vi "BeamProfile_Proc.vi"(5 "Output filepath (For Type Only)":path=path "", 7 "Params.":variant, 8 "error in (no error)":errorcluster, 9 "Dynamic Params queue":refnum<queue>, 10 "Quit_UserEvent":refnum<user-event>, 11 "ControlQueueRef":variant) -> (0 "error out":errorcluster, 2 "Output":variant)   [LabVIEW 2013]
uses:
  Apps_static/ScanParams_SingleLine.ctl
  Files/BinaryHeader.ctl
  ControlDef/QueueRefs.ctl
  ControlDef/LaserCtrl_Method.ctl
  ControlDef/States-AToF.ctl
  <instrlib>/AnalogDiscSDKLv/VIs/DWF_CtrlQueue.ctl
  <instrlib>/AnalogDiscSDKLv/VIs/DWF_State.ctl
  <instrlib>/ESP300/Public/Data/ESP300_State.ctl
  <instrlib>/DG535/Command/DG535_States.ctl
  Hardware/BNC(QuantumComposers)/BNC_States.ctl
  Hardware/FemtoLaser(Legacy)/Laser_Status.ctl
  Hardware/DAQmx(Legacy)/DAQmx_Status.ctl
  ControlDef/Signal.ctl
  ProcessMethods/SignalAverager/ProcessStates.ctl
  Files/WriterState.ctl
  Files/Signal_Segment.ctl
  ControlDef/ProcessingMode.ctl
  Hardware/EPM2000(Legacy)/EPM2K_Status.ctl
  <instrlib>/AnalogDiscSDKLv/VIs/DWF_Signal.ctl
  BeamProfiling_Params.ctl
  <vilib>/Analysis/baseanly.llb/Mean (DBL).vi
  <vilib>/gmath/NumericalOptimization/Nonlinear Curve Fit LM.vi
  <vilib>/gmath/NI_Gmath.lvlib
  <instrlib>/ESP300/ESP300.lvlib
  <instrlib>/DG535/SRS_DG535_Lib.lvlib
  <vilib>/Analysis/NI_AALPro.lvlib
  <instrlib>/AnalogDiscSDKLv/AnalogDiscSDKLv.lvlib
  <vilib>/Analysis/NI_AALBase.lvlib
panel:
  in  "Quit":bool
  out "Photodiode response":sgl[](graph)
  out "Iteration":i32
  out "Filename Indicator":path caption="Filename"
  out "profile fit":dbl[](array[numeric])
  out "R-square":dbl
  out "z0_fit_init.":dbl[](array[numeric])=[0.1, 17.0, 3.0]
  out "best fit parameters":dbl[](array[numeric])
  out "R-Square (w)":dbl
  out "w_fit_init.":dbl[](array[numeric])=[0.0, 1.0, 10.0, 0.01]
  in  "Scan#":u16=1
  out "z (mm)":dbl
  out "raw+fit":cluster{dbl[], "best nonlinear fit":dbl[]}[](graph)
  out "Beam Profile":cluster{dbl[], "best nonlinear fit":dbl[]}[](graph)
  # "radius\n\nfocus at z\n\nrayleigh\nrang"
  # "focus at x\n\nw"
  # "X/y selector stilll has to be added !!"
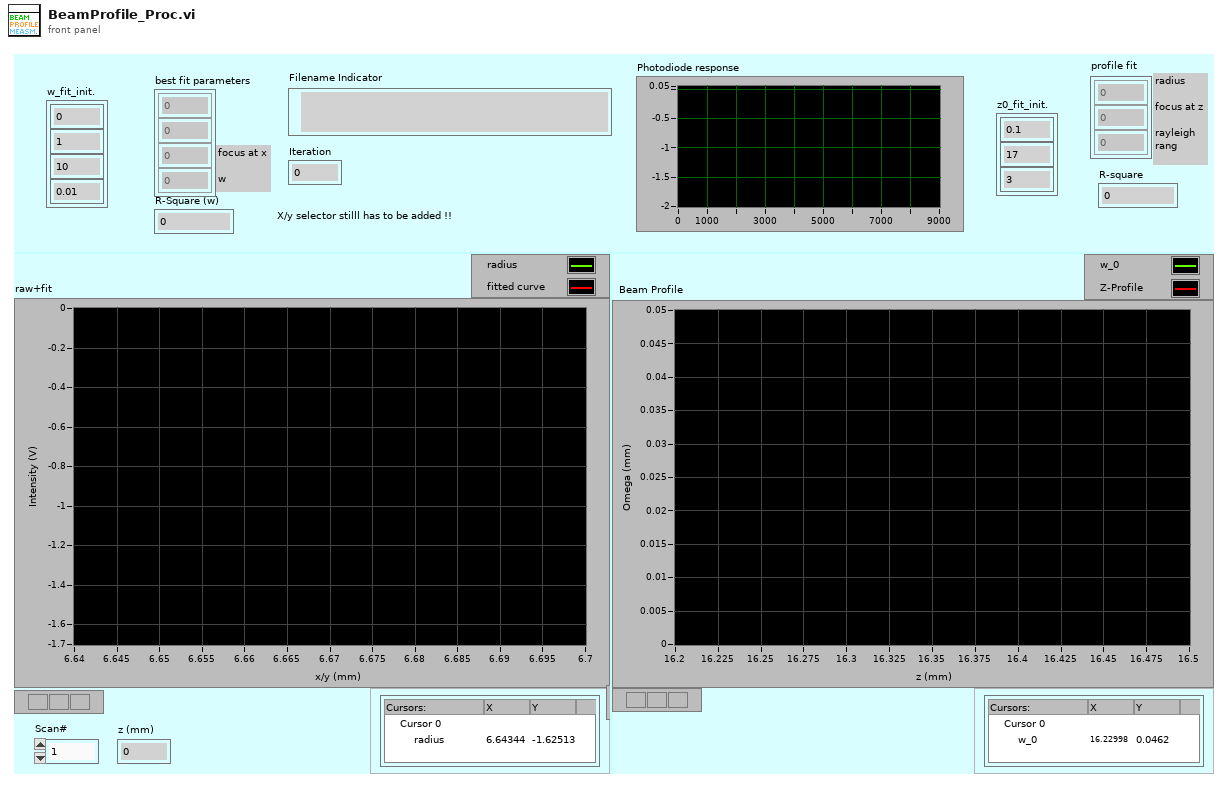
[diagram p1: front panel]
types:
  T1 = typedef "QueueRefs.ctl" = cluster{"LaserCtrlMethod":T2, "Apps":refnum<queue>, "MainDAQCoreQueue":refnum<queue>, "Micos":refnum<queue>, "ESP300":refnum<queue>, "SMC100":refnum<queue>, "SRS DG535":refnum<queue>, "BNC":refnum<queue>, "SDG_ii":refnum<queue>, "NI-USB_DAQmx":refnum<queue>, "ProcCore_CtrlQueue":refnum<queue>, "WriterCtrl":refnum<queue>, "WriterSIG":refnum<queue>, "Feedback":refnum<queue>, "EPM2000":refnum<queue>, "InfoRef":refnum<vi>, "AppsLock":T3, "ProcCore_SignalQueue":refnum<queue>}
  T2 = typedef "LaserCtrl_Method.ctl" = enum16{"SRS_DG535", "BNC", "SDG_II"}
  T3 = typedef "Semaphore RefNum" = refnum<k1>
  T4 = typedef "BeamProfiling_Params.ctl" = cluster{"File Header":T5, "w_fit_init.":dbl[], "z0_fit_init.":dbl[], "LowSpeed":dbl, "HighSpeed":dbl, "x/y?":bool, "IncidentAngle":dbl}
  T5 = typedef "BinaryHeader.ctl" = cluster{"Start Position":dbl[], "StepWidth":dbl[], "Dimension":i32[], "SpecLength":i32}
  T6 = cluster{"State":enum16{"Idle", "Open", "PrepScanParams", "WaitData", "Flush", "ScanResult", "CheckEndCondition", "Close", "Quit", "Refresh_BeamProfileSingle", "Refresh_RayleighRange"}, "Para.":variant}
  T7 = typedef "WriterState.ctl" = cluster{"State":enum16{"Open", "Close", "ChangeFormat", "SetHeader", "QuitProg."}, "Params":variant}
  T8 = typedef "Signal_Segment.ctl" = cluster{"SampleRate":dbl, "TrigDelay":dbl, "SpecLength":dbl, "DAQ_Range":dbl, "Average#":i32, "Position":dbl[], "Spectrum":sgl[], "Calibr.":dbl[], "Pressure":dbl, "Desp_LaserEnergy":dbl, "PI_LaserEnergy":dbl, "Voltages Table":sgl[][], "ProcMode":T9, "Threshold":dbl, "Comment":string, "TickCount":dbl, "Time Stamp":timestamp}
  T9 = typedef "ProcessingMode.ctl" = enum16{"None", "Drop by Threshold", "TDC Simulate", "SetFilter"}
  T10 = cluster{"error":errorcluster, "file path":path, "Save?":bool, "x/y?":bool, "File Header":T5, "Scan#":i32, "ControlRefs":T1, "HighSpeed":dbl, "LowSpeed":dbl, "IncidentAngle":dbl}
  T11 = typedef "ProcessStates.ctl" = enum16{"Initialize", "Normal", "Display", "Write2Buffer", "CalcMzArray", "StartSave", "StopSave", "ConfigChanged", "EndOfLine", "SetFilterParams", "SetGraphsEnable", "SetAcquisitionParams", "ChangeDisplayIncrement", "ChangeRepRate", "SetWriterRef", "Quit", "StartOfLine"}
  T12 = typedef "Signal.ctl" = cluster{"Command":T11, "Params":variant}
  T13 = cluster{"mean":dbl, "Numeric":dbl, "Numeric 2":dbl}[]
  T14 = typedef "ScanParams_SingleLine.ctl" = cluster{"Line Start":dbl[], "Line End":dbl[], "HighSpeed":dbl, "ScanSpeed":dbl, "KeepStill(ms)":u32, "InstruParams":dbl[]}
  T15 = enum16{"Idle", "Open", "PrepScanParams", "WaitData", "Flush", "ScanResult", "CheckEndCondition", "Close", "Quit", "Refresh_BeamProfileSingle", "Refresh_RayleighRange"}
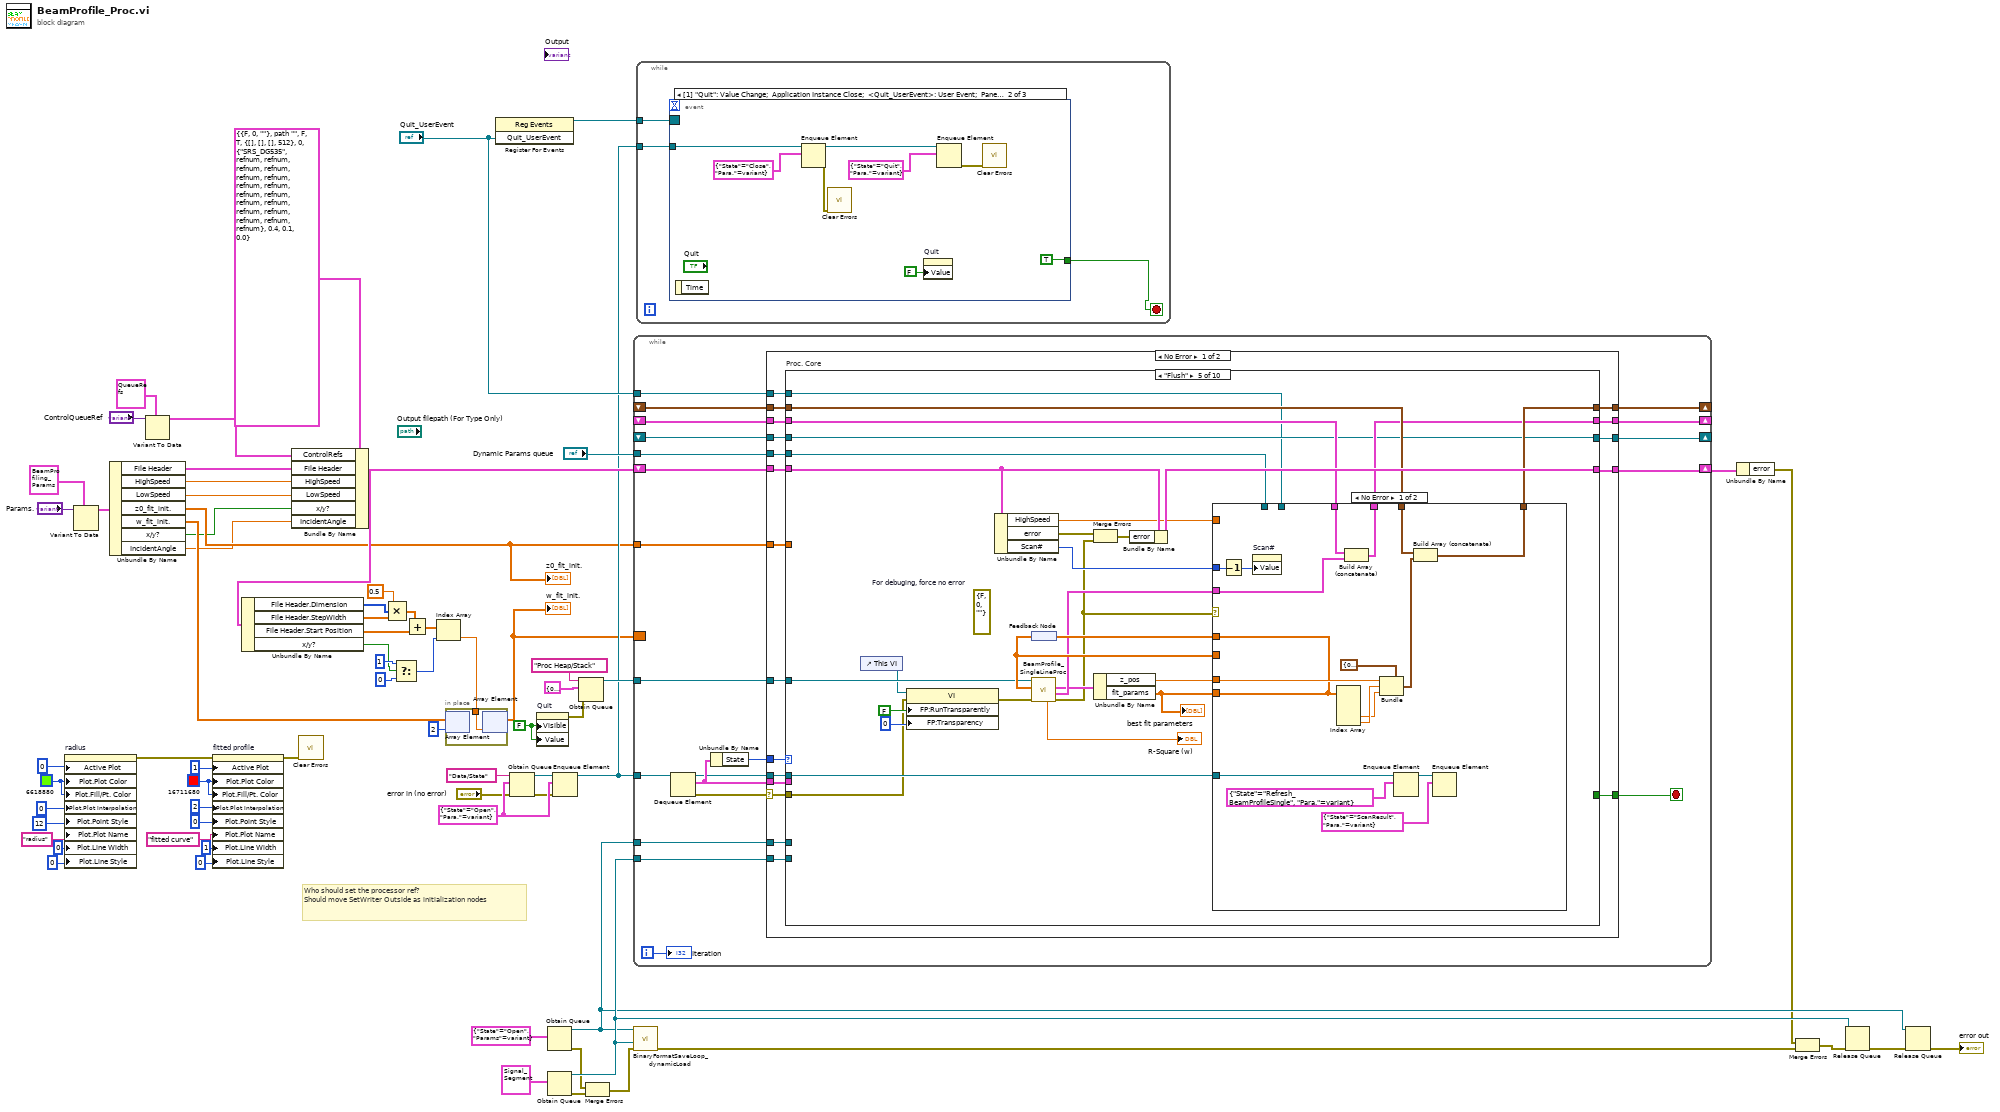
[diagram p0: block diagram]
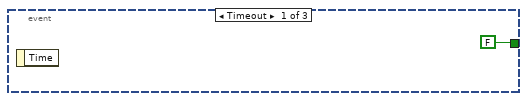
[diagram p2: hidden frame]
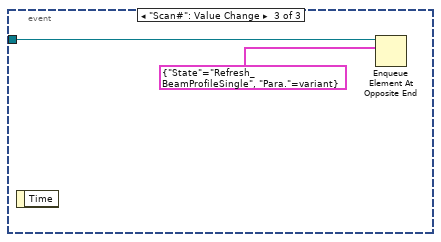
[diagram p3: hidden frame]
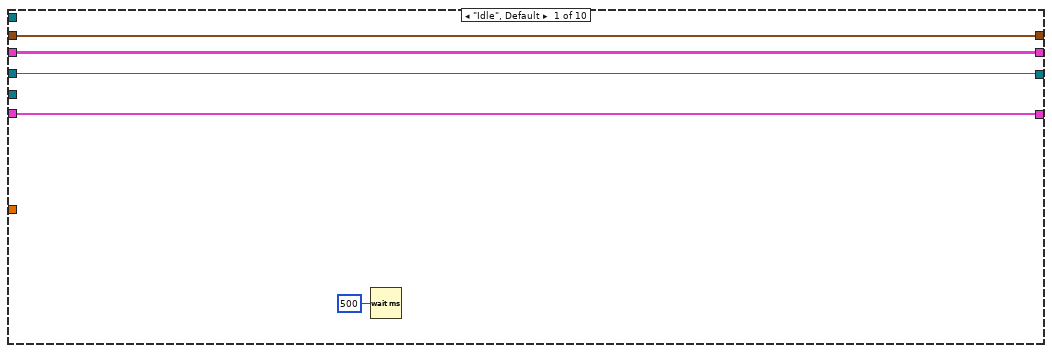
[diagram p4: hidden frame]
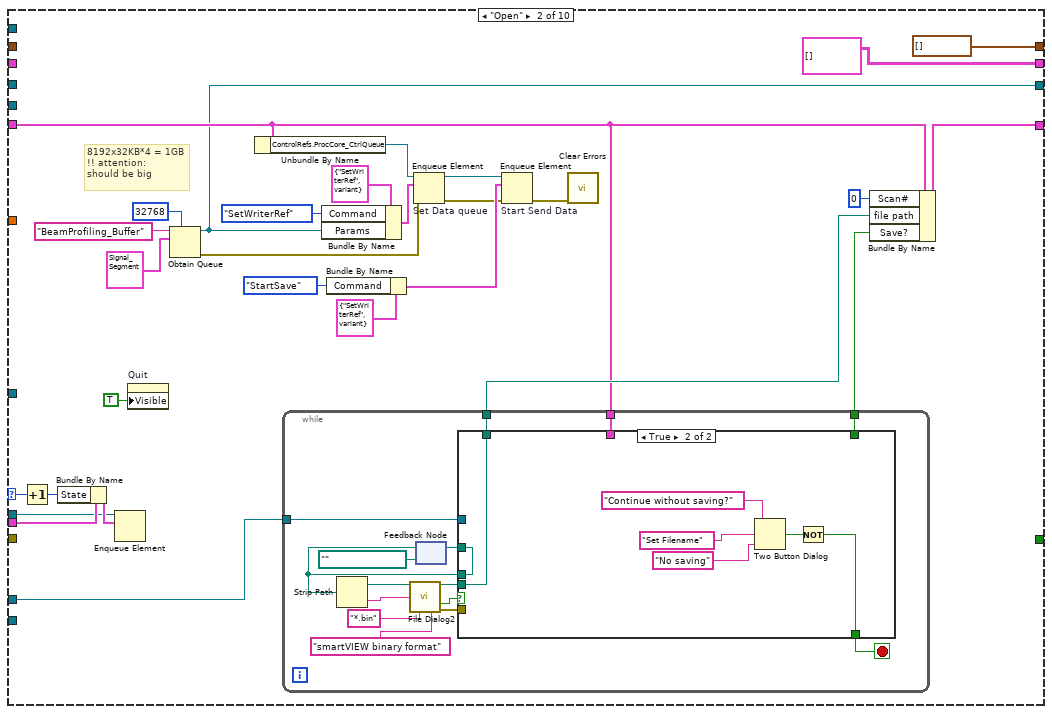
[diagram p5: hidden frame]
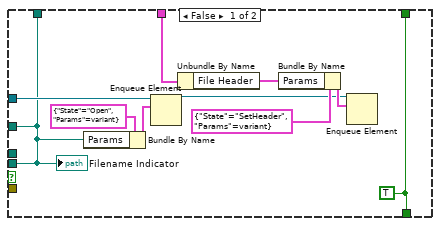
[diagram p6: hidden frame]
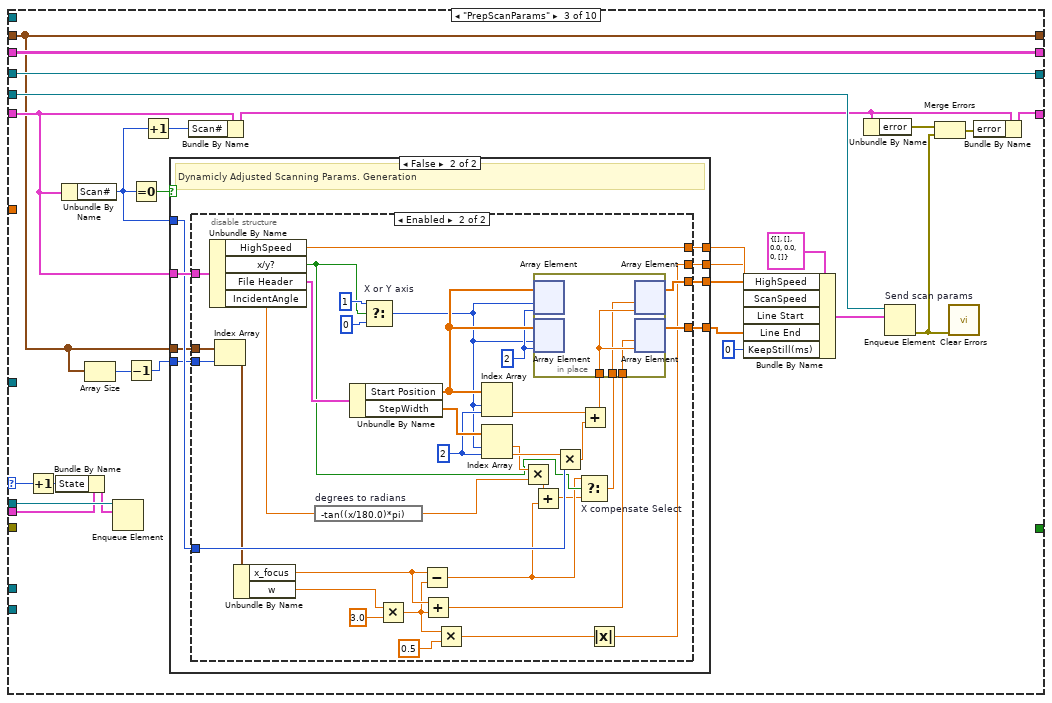
[diagram p7: hidden frame]
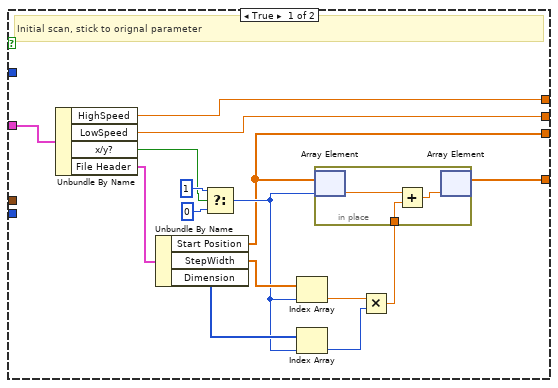
[diagram p8: hidden frame]
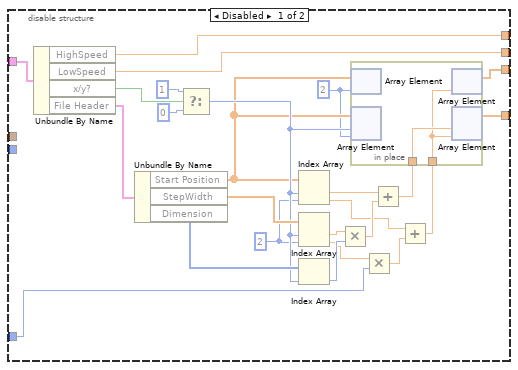
[diagram p9: hidden frame]
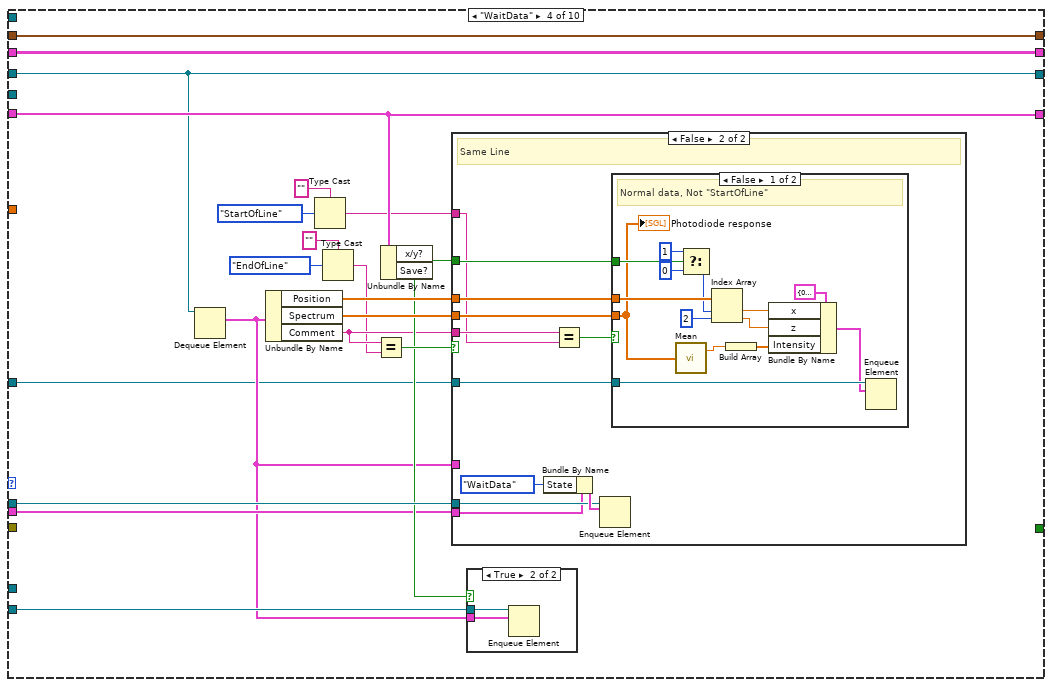
[diagram p10: hidden frame]
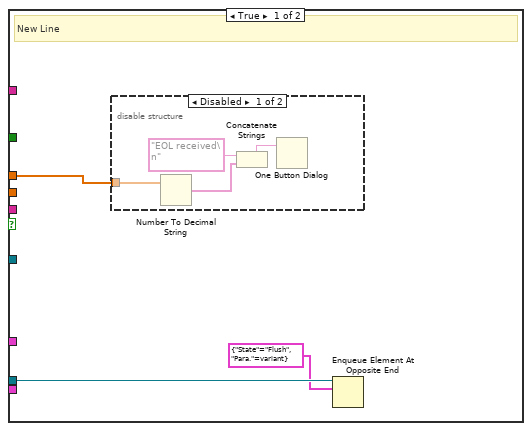
[diagram p12: hidden frame]
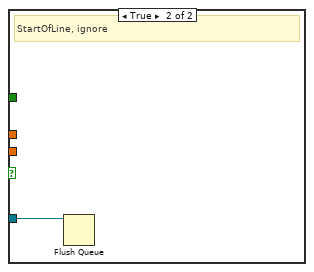
[diagram p14: hidden frame]
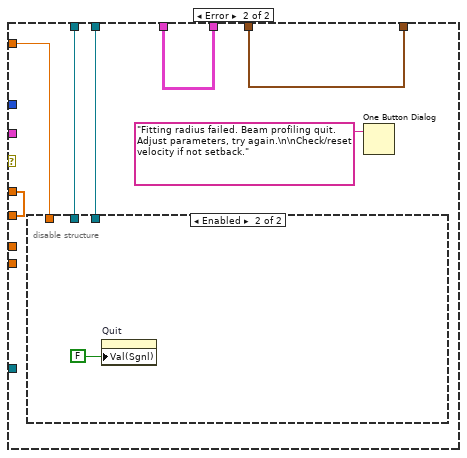
[diagram p15: hidden frame]
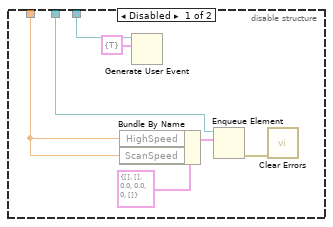
[diagram p16: hidden frame]
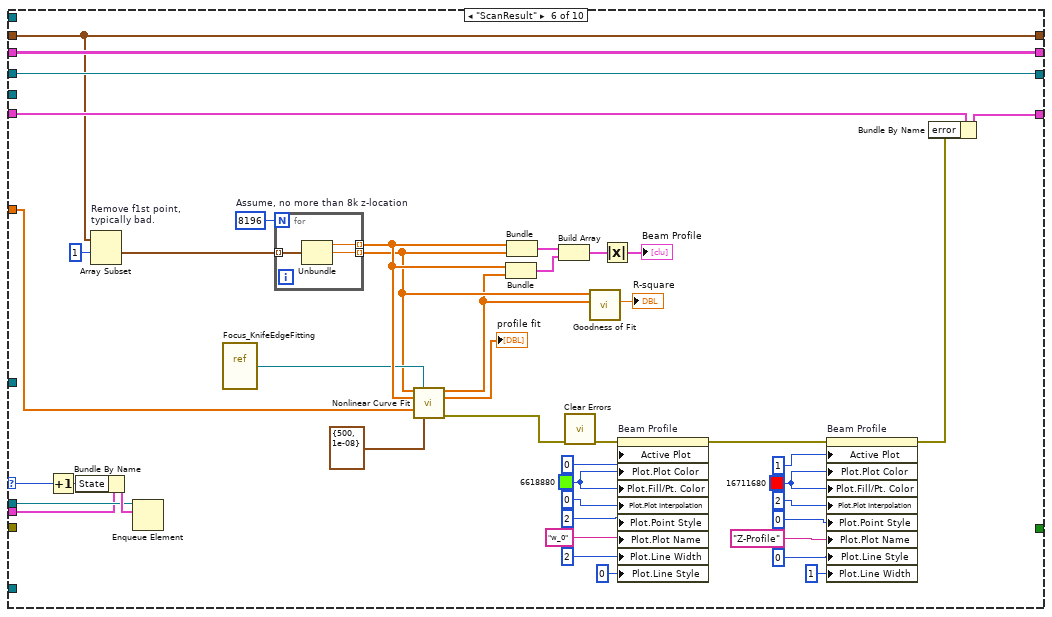
[diagram p17: hidden frame]
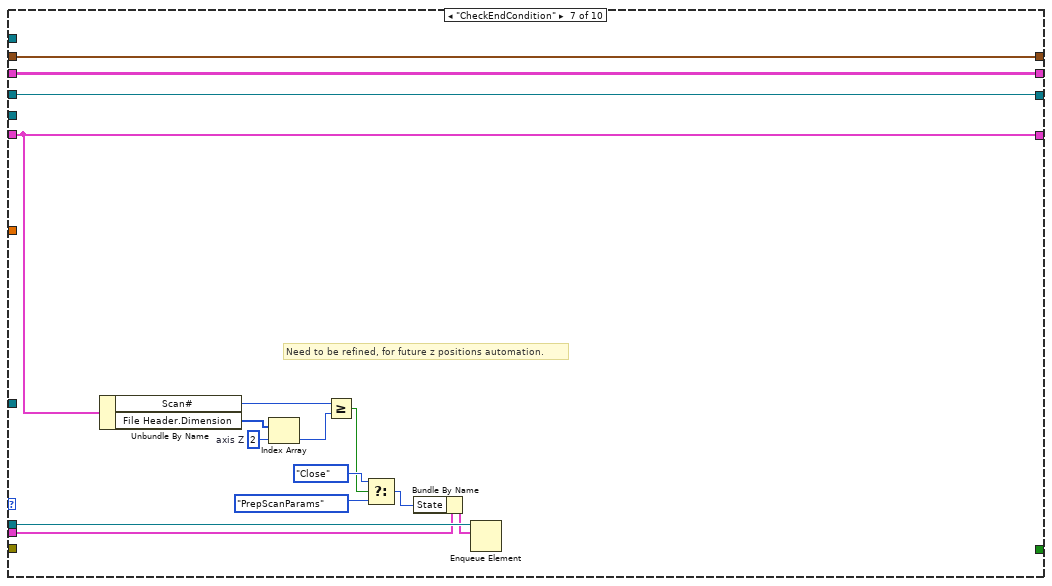
[diagram p18: hidden frame]
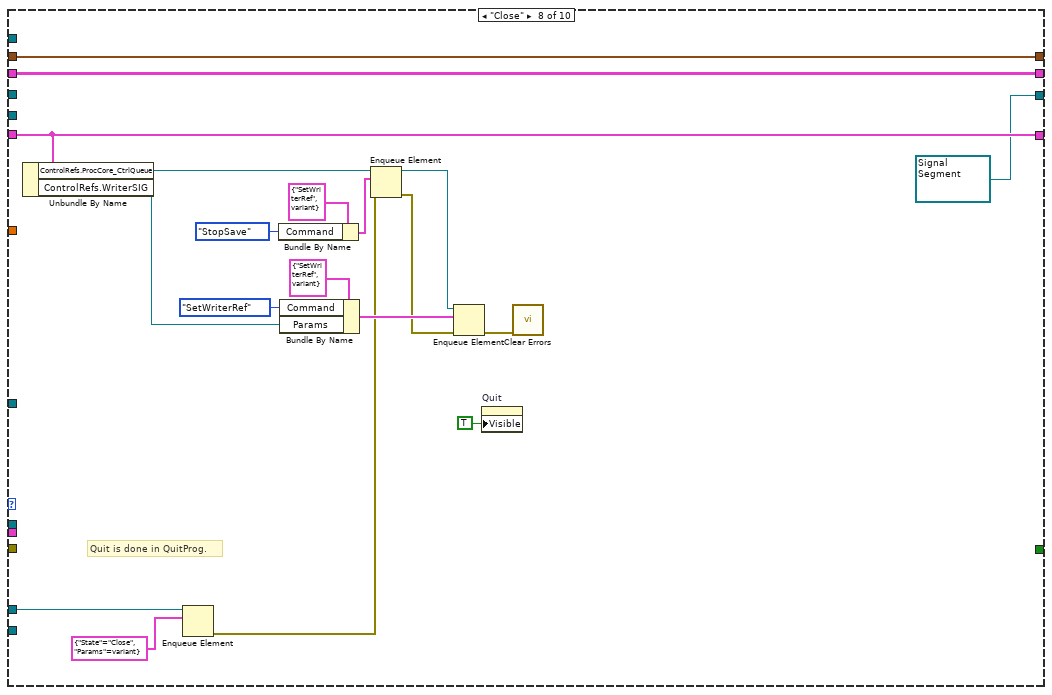
[diagram p19: hidden frame]
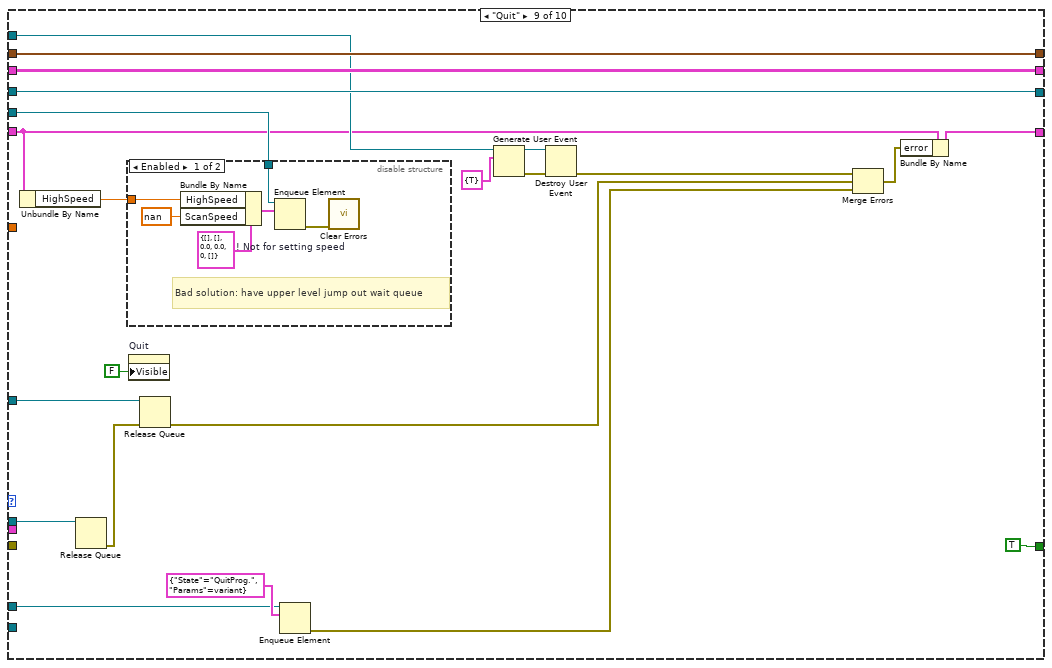
[diagram p20: hidden frame]
diagram:
  w14 = u32 16711680
  w17 = u32 6618880
  w41 = T6 {"State"=enum."Open", "Para."=variant}
  w1 = FALSE ("Visible")
  # "Who should set the processor ref?\nShould move SetWriter Outside as initialization nodes"
  n1 = property on="radius" class="XYGraph (strict)"("Active Plot"=u32 0, "Plot.Plot Color"=w17, "Plot.Fill/Pt. Color"=w17, "Plot.Plot Interpolation"=u8 0 ("Plot.Line Style 2"), "Plot.Point Style"=u8 12 ("Plot.Point Style 2"), "Plot.Plot Name"="radius", "Plot.Line Width"=u8 0, "Plot.Line Style"=u8 0) -> (error out=w12:errorcluster)  [unwired: 2 in, 1 out]
  n2 = Variant To Data(type=T4 {"File Header"={"Start Position"=[], "StepWidth"=[], "Dimension"=[], "SpecLength"=0}, "w_fit_init."=[], "z0_fit_init."=[], "LowSpeed"=0.0, "HighSpeed"=0.0, "x/y?"=FALSE, "IncidentAngle"=0.0} ("BeamProfiling_Params"), Variant="Params.") -> (data=w37:T4)  [unwired: 1 in, 1 out]
  n3 = Unbundle By Name(w37) -> ("File Header"=w35:T5, "HighSpeed"=w34:dbl, "LowSpeed"=w33:dbl, "z0_fit_init."=w31:dbl[], "w_fit_init."=w32:dbl[], "x/y?"=w3:bool, "IncidentAngle"=w2:dbl)
  "z0_fit_init." <- w31
  n4 = Variant To Data(type=T1 {"LaserCtrlMethod"=enum."SRS_DG535", "Apps"=refnum, "MainDAQCoreQueue"=refnum, "Micos"=refnum, "ESP300"=refnum, "SMC100"=refnum, "SRS DG535"=refnum, "BNC"=refnum, "SDG_ii"=refnum, "NI-USB_DAQmx"=refnum, "ProcCore_CtrlQueue"=refnum, "WriterCtrl"=refnum, "WriterSIG"=refnum, "Feedback"=refnum, "EPM2000"=refnum, "InfoRef"=refnum, "AppsLock"=refnum, "ProcCore_SignalQueue"=refnum} ("ControlRefs"), Variant="ControlQueueRef") -> (data=w4:T1)  [unwired: 1 in, 1 out]
  n5 = property on="fitted profile" class="XYGraph (strict)"(error in=w12, "Active Plot"=u32 1, "Plot.Plot Color"=w14, "Plot.Fill/Pt. Color"=w14, "Plot.Plot Interpolation"=u8 2 ("Plot.Line Style"), "Plot.Point Style"=u8 0, "Plot.Plot Name"="fitted curve", "Plot.Line Width"=u8 1, "Plot.Line Style"=u8 0) -> (error out=w13:errorcluster)  [unwired: 1 in, 1 out]
  n6 = Bundle By Name(cluster=T10 {"error"={"status"=FALSE, "code"=0, "source"=""}, "file path"=path "", "Save?"=FALSE, "x/y?"=TRUE, "File Header"={"Start Position"=[], "StepWidth"=[], "Dimension"=[], "SpecLength"=512}, "Scan#"=0, "ControlRefs"={"LaserCtrlMethod"=enum."SRS_DG535", "Apps"=refnum, "MainDAQCoreQueue"=refnum, "Micos"=refnum, "ESP300"=refnum, "SMC100"=refnum, "SRS DG535"=refnum, "BNC"=refnum, "SDG_ii"=refnum, "NI-USB_DAQmx"=refnum, "ProcCore_CtrlQueue"=refnum, "WriterCtrl"=refnum, "WriterSIG"=refnum, "Feedback"=refnum, "EPM2000"=refnum, "InfoRef"=refnum, "AppsLock"=refnum, "ProcCore_SignalQueue"=refnum}, "HighSpeed"=0.4, "LowSpeed"=0.1, "IncidentAngle"=0.0} ("output cluster"), "ControlRefs"=w4, "File Header"=w35, "HighSpeed"=w34, "LowSpeed"=w33, "x/y?"=w3, "IncidentAngle"=w2) -> (w59:T10)
  n7 = Unbundle By Name(w59) -> ("File Header.Dimension"=w53:i32[], "File Header.StepWidth"=w54:dbl[], "File Header.Start Position"=w55:dbl[], "x/y?"=w56:bool)
  n8 = call <vilib>:"Clear Errors.vi"("error in (no error)"=w13) -> ()  [unwired: 6 in, 1 out]
  n9 = Compound Arithmetic op=MULTIPLY(0.5, w53, w54) -> (w51:dbl[])
  n10 = Select(t=1 ("index"), s=w56, f=0 ("index")) -> (s? t:f=w49:i32)
  n11 = Add(x=w51, y=w55) -> (x+y=w50:dbl[])
  n12 = Index Array(array=w50, index=w49) -> (element=w48:dbl)
  n13 = in-place {
    in-place-border: w48 -> [w72]
    n14 = in-place-array #1(w32, 2) -> ()  [unwired: 1 out]
    n15 = in-place-array #1(w72) -> (w36:dbl[])  [unwired: 1 out]
  }
  "w_fit_init." <- w36
  n16 = register-events("Quit_UserEvent") -> (reference out=w62:refnum<event-registration>)  [unwired: 2 in, 1 out]
  n17 = Obtain Queue(name (unnamed)="Data/State", element data type=w41, error in (no error)="error in (no error)") -> (queue out=w42:refnum<queue>, error out=w40:errorcluster)  [unwired: 2 in, 1 out]
  n18 = property on="Quit" class="Bool (strict)"("Visible"=w1, "Value"=w1) -> (error out=w61:errorcluster)  [unwired: 2 in, 1 out]
  n19 = Obtain Queue(element data type=T7 {"State"=enum."Open", "Params"=variant} ("element")) -> (queue out=w45:refnum<queue>, error out=w24:errorcluster)  [unwired: 4 in, 1 out]
  n20 = Obtain Queue(element data type=T8 {"SampleRate"=-1.0, "TrigDelay"=0.0, "SpecLength"=0.0, "DAQ_Range"=0.0, "Average#"=0, "Position"=[], "Spectrum"=[], "Calibr."=[], "Pressure"=-1.0, "Desp_LaserEnergy"=-1.0, "PI_LaserEnergy"=-1.0, "Voltages Table"=[], "ProcMode"=enum."None", "Threshold"=-1.0, "Comment"="", "TickCount"=0.0, "Time Stamp"=timestamp(0 s since 1904-01-01)} ("Signal Segment")) -> (queue out=w46:refnum<queue>, error out=w65:errorcluster)  [unwired: 4 in, 1 out]
  n21 = Enqueue Element(queue=w42, element=w41, error in (no error)=w40) -> (queue out=w38:refnum<queue>)  [unwired: 1 in, 2 out]
  n22 = Obtain Queue(name (unnamed)="Proc Heap/Stack", element data type=cluster{"x":dbl, "z":dbl, "Intensity":sgl[]} {"x"=0.0, "z"=0.0, "Intensity"=[]} ("output cluster"), error in (no error)=w61) -> (queue out=w71:refnum<queue>)  [unwired: 2 in, 2 out]
  n23 = Merge Errors(w24, w65) -> (w25:errorcluster)
  n24 = call "BinaryFormatSaveLoop_dynamicLoad.vi"("data error in"=w25, "data queue in"=w46, "control queue in"=w45) -> ("error out"=w29:errorcluster)  [unwired: 8 in]
  n25 = while {
    shift-right: [w86] -> w64
    shift-left: w59 -> [w93]
    shift-right: [w85] -> _
    shift-left: _ -> [w92]
    tunnel: w38 -> [w91]
    tunnel: w71 -> [w89]
    tunnel: w45 -> [w82]
    tunnel: w46 -> [w81]
    border: w36 -> [_]
    tunnel: "Dynamic Params queue" -> [w80]
    shift-right: [w83] -> _
    shift-left: _ -> [w79]
    shift-right: [w78] -> _
    shift-left: _ -> [w77]
    tunnel: "Quit_UserEvent" -> [w75]
    tunnel: w31 -> [w73]
    i -> [w76]
    stop <- w84 stop-if-true
    n26 = Dequeue Element(queue=w91) -> (queue out=w87:refnum<queue>, element=w88:T6, error out=w90:errorcluster)  [unwired: 2 in, 1 out]
    n27 = Unbundle By Name(w88) -> ("State"=w74:T15)
    n28 = case shown="No Error" w90 {
      selector: w90 -> [w94 _]
      tunnel: w93 -> [w112 w545]
      tunnel: [w111 w545] -> w86
      tunnel: w92 -> [w110 w544]
      tunnel: [w109 w544] -> w85
      tunnel: w89 -> [w108 _]
      tunnel: w74 -> [w107 _]
      tunnel: w88 -> [w106 _]
      tunnel: w87 -> [w105 _]
      tunnel: [w104 TRUE] -> w84
      tunnel: [w103 w542] -> w83
      tunnel: w82 -> [w102 _]
      tunnel: w81 -> [w101 _]
      tunnel: w80 -> [w100 _]
      tunnel: w79 -> [w99 w542]
      tunnel: [w98 w541] -> w78
      tunnel: w77 -> [w97 w541]
      tunnel: w75 -> [w96 _]
      tunnel: w73 -> [w95 _]
      frame No Error {
        n29 = case "Proc. Core" shown="\"Flush\"" w107 {
          selector: w107 -> [_ w133 w190 _ _ w451 _ _ _ _]
          tunnel: w112 -> [w117 w138 w204 w313 w372 w456 w469 w487 w495 w535]
          tunnel: [w117 w145 w187 w313 w381 w426 w469 w487 w502 w535] -> w111
          tunnel: [w116 T13 [] ("appended array") w180 w318 w379 w415 w474 w493 w515 w534] -> w109
          tunnel: w110 -> [w116 _ w180 w318 w380 w415 w474 w493 w515 w534]
          tunnel: w108 -> [_ _ _ w298 w368 _ _ _ w513 _]
          tunnel: w106 -> [_ w135 w192 w308 _ w452 w467 _ _ _]
          tunnel: w105 -> [_ w134 w193 w317 w358 w453 w468 _ w503 w536]
          tunnel: [_ _ _ _ _ _ _ _ TRUE _] -> w104
          tunnel: [w114 cluster{dbl[], dbl[]}[][] [] w188 w307 w373 w423 w466 w485 w510 w533] -> w103
          tunnel: w102 -> [_ w143 _ _ _ _ _ w492 w511 _]
          tunnel: w101 -> [_ _ _ w312 _ _ _ _ _ _]
          tunnel: w100 -> [_ _ w195 _ w362 _ _ _ w497 _]
          tunnel: w99 -> [w114 _ w188 w307 w374 w423 w466 w485 w510 w533]
          tunnel: [w113 w129 w182 w305 w369 w421 w465 refnum<queue> refnum ("Data") w509 w532] -> w98
          tunnel: w97 -> [w113 _ w182 w305 w369 w421 w465 _ w509 w532]
          tunnel: w96 -> [_ _ _ _ w363 _ _ _ w508 _]
          tunnel: w95 -> [_ _ _ _ _ w420 _ _ _ _]
          tunnel: w94 -> [_ _ _ _ w357 _ _ _ _ _]
          frame "Idle", Default {
            n30 = Wait (ms)(milliseconds to wait=u32 500) -> ()  [unwired: 1 out]
          }
          frame "Open" {
            # "8192x32KB*4 = 1GB\n!! attention:\nshould be big"
            n31 = Increment(x=w133) -> (x+1=w136:T15)
            n32 = Bundle By Name(cluster=w135, "State"=w136) -> (w137:T6)
            n33 = Enqueue Element(queue=w134, element=w137) -> ()  [unwired: 2 in, 3 out]
            n34 = property on="Quit" class="Bool (strict)"("Visible"=TRUE) -> ()  [unwired: 2 in, 2 out]
            n35 = Obtain Queue(max queue size (-1, unlimited)=32768, name (unnamed)="BeamProfiling_Buffer", element data type=T8 {"SampleRate"=0.0, "TrigDelay"=0.0, "SpecLength"=0.0, "DAQ_Range"=0.0, "Average#"=0, "Position"=[], "Spectrum"=[], "Calibr."=[], "Pressure"=0.0, "Desp_LaserEnergy"=0.0, "PI_LaserEnergy"=0.0, "Voltages Table"=[], "ProcMode"=enum."None", "Threshold"=0.0, "Comment"="", "TickCount"=0.0, "Time Stamp"=timestamp(0 s since 1904-01-01)} ("Signal Segment")) -> (queue out=w129:refnum<queue>, error out=w128:errorcluster)  [unwired: 2 in, 1 out]
            n36 = Unbundle By Name(w138) -> ("ControlRefs.ProcCore_CtrlQueue"=w130:refnum<queue>)
            n37 = while {
              tunnel: [w151] -> w144
              tunnel: w143 -> [w150]
              tunnel: [w149] -> w142
              tunnel: w138 -> [w148]
              stop <- w152 stop-if-true
              n38 = feedback #2(path "" ("selected path")) -> (w160:path)
              n39 = Strip Path(path=w160) -> (stripped path=w157:path, name=w158:string)
              n40 = call "File Dialog2"("start path"=w157, "default name"=w158, "pattern (all files)"="*.bin", "pattern label"="smartVIEW binary format") -> ("selected path"=w156:path, "cancelled"=w153:bool, "error out"=w154:errorcluster)  [unwired: 8 in, 1 out]
              n41 = case shown="True" w153 {
                tunnel: w150 -> [w171 _]
                tunnel: w156 -> [w164 w175]
                tunnel: w154 -> [_ _]
                tunnel: [w164 w176] -> w159
                tunnel: w160 -> [_ w176]
                tunnel: [w165 w174] -> w152
                tunnel: [w164 w175] -> w151
                tunnel: [w165 _] -> w149
                tunnel: w148 -> [w162 _]
                frame False {
                  w165 = TRUE
                  n42 = Bundle By Name(cluster=T7 {"State"=enum."Open", "Params"=variant} ("element"), "Params"=w164) -> (w169:T7)
                  n43 = Enqueue Element(queue=w171, element=w169) -> (queue out=w166:refnum<queue>)  [unwired: 2 in, 2 out]
                  n44 = Unbundle By Name(w162) -> ("File Header"=w163:T5)
                  n45 = Bundle By Name(cluster=T7 {"State"=enum."SetHeader", "Params"=variant} ("element"), "Params"=w163) -> (w168:T7)
                  n46 = Enqueue Element(queue=w166, element=w168) -> ()  [unwired: 2 in, 3 out]
                  "Filename Indicator" <- w164
                }
                frame True {
                  n47 = Two Button Dialog(message="Continue without saving?", 1:"No saving" ("F button name (\"Cancel\")"), 2:"Set Filename" ("T button name (\"OK\")")) -> (T button?=w177:bool)
                  n48 = Not(x=w177) -> (.not. x?=w174:bool)
                }
              }
              n49 = feedback-in #2(w159) -> ()
            }
            n50 = Bundle By Name(cluster=T12 {"Command"=enum."SetWriterRef", "Params"=variant} ("element"), "Command"=ProcessStates."SetWriterRef", "Params"=w129) -> (w140:T12)
            n51 = Bundle By Name(cluster=T12 {"Command"=enum."SetWriterRef", "Params"=variant} ("element"), "Command"=ProcessStates."StartSave") -> (w125:T12)
            n52 = Enqueue Element "Set Data queue"(queue=w130, element=w140, error in (no error)=w128) -> (queue out=w123:refnum<queue>, error out=w122:errorcluster)  [unwired: 1 in, 1 out]
            n53 = Enqueue Element "Start Send Data"(queue=w123, element=w125, error in (no error)=w122) -> (error out=w121:errorcluster)  [unwired: 1 in, 2 out]
            n54 = call <vilib>:"Clear Errors.vi"("error in (no error)"=w121) -> ()  [unwired: 6 in, 1 out]
            n55 = Bundle By Name(cluster=w138, "Scan#"=0, "file path"=w144, "Save?"=w142) -> (w145:T10)
          }
          frame "PrepScanParams" {
            n56 = Increment(x=w190) -> (x+1=w189:T15)
            n57 = Bundle By Name(cluster=w192, "State"=w189) -> (w191:T6)
            n58 = Unbundle By Name(w204) -> ("Scan#"=w196:i32)
            n59 = Array Size(array=w180) -> (size(s)=w181:i32)
            n60 = Enqueue Element(queue=w193, element=w191) -> ()  [unwired: 2 in, 3 out]
            n61 = Decrement(x=w181) -> (x-1=w179:i32)
            n62 = Equal To 0?(x=w196) -> (x = 0?=w205:bool)
            n63 = Increment(x=w196) -> (x+1=w203:i32)
            n64 = case shown="False" w205 {
              tunnel: w204 -> [w220 w231]
              tunnel: [w206 w226] -> w201
              tunnel: [w211 w230] -> w200
              tunnel: [w210 w229] -> w199
              tunnel: [w209 w228] -> w198
              tunnel: w196 -> [_ w227]
              tunnel: w180 -> [_ w225]
              tunnel: w179 -> [_ w224]
              frame True {
                # "Initial scan, stick to orignal parameter"
                n65 = Unbundle By Name(w220) -> ("HighSpeed"=w210:dbl, "LowSpeed"=w209:dbl, "x/y?"=w207:bool, "File Header"=w215:T5)
                n66 = Unbundle By Name(w215) -> ("Start Position"=w206:dbl[], "StepWidth"=w218:dbl[], "Dimension"=w219:i32[])
                n67 = Select(t=1 ("index"), s=w207, f=0 ("index")) -> (s? t:f=w212:i32)
                n68 = Index Array(array=w218, index=w212) -> (element=w217:dbl)
                n69 = Index Array(array=w219, index=w212) -> (element=w216:i32)
                n70 = Multiply(x=w217, y=w216) -> (x*y=w208:dbl)
                n71 = in-place {
                  in-place-border: w208 -> [w222]
                  n72 = in-place-array #3(w206, w212) -> (w223:dbl)
                  n73 = Add(x=w223, y=w222) -> (x+y=w221:dbl)
                  n74 = in-place-array #3(w221) -> (w211:dbl[])  [unwired: 1 out]
                }
              }
              frame False {
                # "Dynamicly Adjusted Scanning Params. Generation"
                n75 = disable-structure shown="Enabled" {
                  disable-tunnel: w231 -> [w256 w294]
                  disable-tunnel: [w243 w289] -> w230
                  disable-tunnel: [w242 w288] -> w229
                  disable-tunnel: [w241 w259] -> w228
                  disable-tunnel: w227 -> [w235 w282]
                  disable-tunnel: [w232 w280] -> w226
                  disable-tunnel: w225 -> [_ w277]
                  disable-tunnel: w224 -> [_ w276]
                  frame Disabled {
                    w240 = 2 ("index")
                    w233 = 2
                    n76 = Unbundle By Name(w256) -> ("HighSpeed"=w242:dbl, "LowSpeed"=w241:dbl, "x/y?"=w246:bool, "File Header"=w249:T5)
                    n77 = Unbundle By Name(w249) -> ("Start Position"=w234:dbl[], "StepWidth"=w254:dbl[], "Dimension"=w255:i32[])
                    n78 = Select(t=1 ("index"), s=w246, f=0 ("index")) -> (s? t:f=w244:i32)
                    n79 = Index Array(array=w234, index #1=w244, index #2=w240) -> (element #1=w253:dbl, element #2=w237:dbl)
                    n80 = Index Array(array=w254, index #1=w244, index #2=w240) -> (element #1=w251:dbl, element #2=w239:dbl)
                    n81 = Index Array(array=w255, index=w244) -> (element=w250:i32)
                    n82 = Multiply(x=w251, y=w250) -> (x*y=w252:dbl)
                    n83 = Multiply(x=w239, y=w235) -> (x*y=w238:dbl)
                    n84 = Add(x=w253, y=w252) -> (x+y=w245:dbl)
                    n85 = Add(x=w237, y=w238) -> (x+y=w236:dbl)
                    n86 = in-place {
                      in-place-border: w245 -> [w258]
                      in-place-border: w236 -> [w257]
                      n87 = in-place-array #4(w234, w233) -> ()  [unwired: 1 out]
                      n88 = in-place-array #5(w234, w244, w233) -> ()  [unwired: 2 out]
                      n89 = in-place-array #4(w257) -> (w232:dbl[])  [unwired: 1 out]
                      n90 = in-place-array #5(w258, w257) -> (w243:dbl[])  [unwired: 2 out]
                    }
                  }
                  frame Enabled {
                    w287 = 2 ("index")
                    w279 = 2
                    n91 = Unbundle By Name(w294) -> ("HighSpeed"=w288:dbl, "x/y?"=w263:bool, "File Header"=w292:T5, "IncidentAngle"=w266:dbl)
                    n92 = Index Array(array=w277, index=w276) -> (element=w275:cluster{"z_pos":dbl, "w":dbl, "x_focus":dbl})
                    n93 = Unbundle By Name(w275) -> ("x_focus"=w274:dbl, "w"=w273:dbl)
                    n94 = expression code="-tan((x/180.0)*pi)" "degrees to radians"(w266) -> (w267:dbl)
                    n95 = Unbundle By Name(w292) -> ("Start Position"=w281:dbl[], "StepWidth"=w293:dbl[])
                    n96 = Select "X or Y axis"(t=1 ("index"), s=w263, f=0 ("index")) -> (s? t:f=w278:i32)
                    n97 = Multiply(x=w273, y=3.0) -> (x*y=w270:dbl)
                    n98 = Subtract(x=w274, y=w270) -> (x-y=w261:dbl)
                    n99 = Add(x=w274, y=w270) -> (x+y=w271:dbl)
                    n100 = Multiply(x=w270, y=0.5) -> (x*y=w268:dbl)
                    n101 = Index Array(array=w281, index #1=w278, index #2=w287) -> (element #2=w284:dbl)  [unwired: 1 out]
                    n102 = Index Array(array=w293, index #1=w278, index #2=w287) -> (element #1=w265:dbl, element #2=w286:dbl)
                    n103 = Multiply(x=w265, y=w267) -> (x*y=w262:dbl)
                    n104 = Add(x=w262, y=w261) -> (x+y=w260:dbl)
                    n105 = Multiply(x=w286, y=w282) -> (x*y=w285:dbl)
                    n106 = Select "X compensate Select"(t=w261, s=w263, f=w260) -> (s? t:f=w264:dbl)
                    n107 = Add(x=w284, y=w285) -> (x+y=w283:dbl)
                    n108 = in-place {
                      in-place-border: w283 -> [w297]
                      in-place-border: w264 -> [w296]
                      in-place-border: w271 -> [w295]
                      n109 = in-place-array #6(w281, w278, w279) -> ()  [unwired: 2 out]
                      n110 = in-place-array #7(w281, w278, w279) -> ()  [unwired: 2 out]
                      n111 = in-place-array #6(w296, w297) -> (w280:dbl[])  [unwired: 2 out]
                      n112 = in-place-array #7(w295, w297) -> (w289:dbl[])  [unwired: 2 out]
                    }
                    n113 = Absolute Value(x=w268) -> (abs(x)=w259:dbl)
                  }
                }
              }
            }
            n114 = Bundle By Name(cluster=w204, "Scan#"=w203) -> (w183:T10)
            n115 = Bundle By Name(cluster=T14 {"Line Start"=[], "Line End"=[], "HighSpeed"=0.0, "ScanSpeed"=0.0, "KeepStill(ms)"=0, "InstruParams"=[]}, "HighSpeed"=w199, "ScanSpeed"=w198, "Line Start"=w201, "Line End"=w200, "KeepStill(ms)"=u32 0 ("Wait(ms)")) -> (w194:T14)
            n116 = Unbundle By Name(w183) -> ("error"=w184:errorcluster)
            n117 = Enqueue Element "Send scan params"(queue=w195, element=w194) -> (error out=w185:errorcluster)  [unwired: 2 in, 2 out]
            n118 = Merge Errors(w184, w185) -> (w186:errorcluster)
            n119 = call <vilib>:"Clear Errors.vi"("error in (no error)"=w185) -> ()  [unwired: 6 in, 1 out]
            n120 = Bundle By Name(cluster=w183, "error"=w186) -> (w187:T10)
          }
          frame "WaitData" {
            n121 = Dequeue Element(queue=w305) -> (element=w306:T8)  [unwired: 2 in, 3 out]
            n122 = Unbundle By Name(w306) -> ("Position"=w314:dbl[], "Spectrum"=w315:sgl[], "Comment"=w310:string)
            n123 = Type Cast(type="", x=ProcessStates."StartOfLine") -> (*(type *) &x=w299:string)
            n124 = Type Cast(type="", x=ProcessStates."EndOfLine") -> (*(type *) &x=w302:string)
            n125 = Equal?(x=w310, y=w302) -> (x = y?=w316:bool)
            n126 = Unbundle By Name(w313) -> ("x/y?"=w309:bool, "Save?"=w311:bool)
            n127 = case shown="False" w316 {
              tunnel: w317 -> [w323 w332]
              tunnel: w298 -> [_ w328]
              tunnel: w315 -> [_ w338]
              tunnel: w314 -> [w321 w337]
              tunnel: w306 -> [_ _]
              tunnel: w310 -> [_ w336]
              tunnel: w309 -> [_ w334]
              tunnel: w308 -> [_ w331]
              tunnel: w299 -> [_ w329]
              frame True {
                # "New Line"
                n128 = disable-structure shown="Disabled" {
                  disable-tunnel: w321 -> [w326 _]
                  frame Disabled {
                    n129 = Number To Decimal String(number=w326) -> (decimal integer string=w324:string[])  [unwired: 1 in]
                    n130 = Concatenate Strings("EOL received\n" ("message"), w324) -> (w325:string)
                    n131 = One Button Dialog(message=w325) -> ()  [unwired: 1 in, 1 out]
                  }
                  frame Enabled {
                  }
                }
                n132 = Enqueue Element At Opposite End(queue=w323, element=T6 {"State"=enum."Flush", "Para."=variant}) -> ()  [unwired: 2 in, 3 out]
              }
              frame False {
                # "Same Line"
                n133 = Bundle By Name(cluster=w331, "State"=T15."WaitData") -> (w333:T6)
                n134 = Equal?(x=w336, y=w329) -> (x = y?=w335:bool)
                n135 = Enqueue Element(queue=w332, element=w333) -> ()  [unwired: 2 in, 3 out]
                n136 = case shown="False" w335 {
                  tunnel: w328 -> [w352 w353]
                  tunnel: w338 -> [w342 _]
                  tunnel: w337 -> [w351 _]
                  tunnel: w334 -> [w343 _]
                  frame False {
                    # "Normal data, Not \"StartOfLine\""
                    n137 = call-poly <vilib>:"Mean.vi"("X"=w342) -> ("mean"=w339:dbl)  [unwired: 1 out]
                    n138 = Select(t=1 ("index"), s=w343, f=0 ("index")) -> (s? t:f=w346:i32)
                    n139 = Index Array(array=w351, index #1=w346, index #2=2 ("index")) -> (element #1=w340:dbl, element #2=w350:dbl)
                    n140 = Build Array(w339) -> (w341:dbl[])
                    n141 = Bundle By Name(cluster=cluster{"x":dbl, "z":dbl, "Intensity":sgl[]} {"x"=0.0, "z"=0.0, "Intensity"=[]} ("element"), "x"=w340, "z"=w350, "Intensity"=w341) -> (w345:cluster{"x":dbl, "z":dbl, "Intensity":sgl[]})
                    n142 = Enqueue Element(queue=w352, element=w345) -> ()  [unwired: 2 in, 3 out]
                    "Photodiode response" <- w342
                  }
                  frame True {
                    # "StartOfLine, ignore"
                    n143 = Flush Queue(queue=w353) -> ()  [unwired: 1 in, 3 out]
                  }
                }
              }
            }
            n144 = case shown="True" w311 {
              tunnel: w312 -> [_ w320]
              tunnel: w306 -> [_ w319]
              frame False {
              }
              frame True {
                n145 = Enqueue Element(queue=w320, element=w319) -> ()  [unwired: 2 in, 3 out]
              }
            }
          }
          frame "Flush" {
            (unwired) errorcluster {"status"=FALSE, "code"=0, "source"=""}  # For debuging, force no error
            n146 = control-ref of="This VI"() -> (w367:refnum<vi>)
            n147 = property class="VI"(reference=w367, error in=w357, "FP:RunTransparently"=FALSE ("Front Panel Window:Run VI Transparently"), "FP:Transparency"=u8 0 ("Front Panel Window:Transparency")) -> (error out=w364:errorcluster)  [unwired: 1 out]
            n148 = Unbundle By Name(w372) -> ("HighSpeed"=w355:dbl, "error"=w371:errorcluster, "Scan#"=w356:i32)
            n149 = feedback #8() -> (w376:dbl[])
            n150 = call "BeamProfile_SingleLineProc.vi"("error in"=w364, "initial parameters"=w376, "data queue in"=w368) -> ("error out"=w354:errorcluster, "Points/Fitted Curve"=w375:cluster{dbl[], dbl[]}[], "fit params"=w360:cluster{"z_pos":dbl, "fit_params":dbl[]}, "R-square"=→"R-Square (w)":dbl)  [unwired: 5 in]
            n151 = Merge Errors(w371, w354) -> (w370:errorcluster)
            n152 = Unbundle By Name(w360) -> ("z_pos"=w361:dbl, "fit_params"=w359:dbl[])
            "best fit parameters" <- w359
            n153 = Bundle By Name(cluster=w372, "error"=w370) -> (w381:T10)
            n154 = case shown="No Error" w354 {
              tunnel: w380 -> [w398 w405]
              tunnel: [w397 w405] -> w379
              tunnel: [w389 w404] -> w377
              tunnel: w376 -> [_ w404]
              tunnel: w375 -> [w392 _]
              tunnel: w374 -> [w393 w403]
              tunnel: [w384 w403] -> w373
              tunnel: w363 -> [_ w399]
              tunnel: w362 -> [_ w401]
              tunnel: w361 -> [w390 _]
              tunnel: w359 -> [w389 _]
              tunnel: w358 -> [w388 _]
              tunnel: w356 -> [w383 _]
              tunnel: w355 -> [_ w400]
              frame No Error {
                n155 = Decrement(x=w383) -> (x-1=w382:i32)
                n156 = property on="Scan#" class="DigNum (strict)"("Value"=w382) -> ()  [unwired: 2 in, 2 out]
                n157 = Index Array(array=w389) -> (element #3=w394:dbl, element #4=w395:dbl)  [unwired: 4 in, 2 out]
                n158 = Build Array (concatenate)(w393, w392) -> (w384:cluster{dbl[], dbl[]}[][])
                n159 = Bundle(cluster=cluster{"z_pos":dbl, "w":dbl, "x_focus":dbl} {"z_pos"=0.0, "w"=0.0, "x_focus"=0.0}, "z_pos"=w390, "w"=w395, "x_focus"=w394) -> (w396:cluster{"z_pos":dbl, "w":dbl, "x_focus":dbl})
                n160 = Enqueue Element(queue=w388, element=T6 {"State"=enum."Refresh_BeamProfileSingle", "Para."=variant}) -> (queue out=w387:refnum<queue>)  [unwired: 2 in, 2 out]
                n161 = Build Array (concatenate)(w398, w396) -> (w397:cluster{"z_pos":dbl, "w":dbl, "x_focus":dbl}[])
                n162 = Enqueue Element(queue=w387, element=T6 {"State"=enum."ScanResult", "Para."=variant}) -> ()  [unwired: 2 in, 3 out]
              }
              frame Error {
                n163 = disable-structure shown="Enabled" {
                  disable-tunnel: w401 -> [w412 _]
                  disable-tunnel: w400 -> [w408 _]
                  disable-tunnel: w399 -> [w406 _]
                  frame Disabled {
                    n164 = Bundle By Name(cluster=T14 {"Line Start"=[], "Line End"=[], "HighSpeed"=0.0, "ScanSpeed"=0.0, "KeepStill(ms)"=0, "InstruParams"=[]} ("element"), "HighSpeed"=w408, "ScanSpeed"=w408) -> (w409:T14)
                    n165 = Generate User Event(user event=w406, event data cluster=cluster{"Quit":bool} {"Quit"=TRUE} ("event data")) -> ()  [unwired: 2 in, 2 out]
                    n166 = Enqueue Element(queue=w412, element=w409) -> (error out=w410:errorcluster)  [unwired: 2 in, 2 out]
                    n167 = call <vilib>:"Clear Errors.vi"("error in (no error)"=w410) -> ()  [unwired: 6 in, 1 out]
                  }
                  frame Enabled {
                    n168 = property on="Quit" class="Bool (strict)"("Val(Sgnl)"=FALSE ("Quit")) -> ()  [unwired: 2 in, 2 out]
                  }
                }
                n169 = One Button Dialog(message="Fitting radius failed. Beam profiling quit. Adjust parameters, try again.\n\nCheck/reset velocity if not setback.") -> ()  [unwired: 1 in, 1 out]
              }
            }
            n170 = feedback-in #8(w377) -> ()
          }
          frame "ScanResult" {
            w422 = 8196  # Assume, no more than 8k z-location
            w431 = u32 16711680
            w433 = u32 6618880
            n171 = Increment(x=w451) -> (x+1=w454:T15)
            n172 = Bundle By Name(cluster=w452, "State"=w454) -> (w455:T6)
            n173 = Array Subset "Remove f1st point, \ntypically bad."(array=w415, index=1) -> (w416:cluster{"z_pos":dbl, "w":dbl, "x_focus":dbl}[])  [unwired: 1 in]
            n174 = Enqueue Element(queue=w453, element=w455) -> ()  [unwired: 2 in, 3 out]
            n175 = vi-ref "Focus_KnifeEdgeFitting.vi"() -> (w443:refnum<vi>)
            n176 = for {
              N: w422 -> [_]
              tunnel: w416 -> [w459] mode=indexing
              tunnel: [w458] -> w445 mode=indexing
              tunnel: [w457] -> w418 mode=indexing
              n177 = Unbundle(w459) -> ("z_pos"=w458:dbl, "w"=w457:dbl)  [unwired: 1 out]
            }
            n178 = call-poly <vilib>:"Nonlinear Curve Fit.vi"("Y"=w418, "f(x,a)"=w443, "X"=w445, "initial parameters"=w420, "termination"=cluster{"max iteration":i32, "tolerance":dbl} {"max iteration"=500, "tolerance"=1e-08}) -> ("best nonlinear fit"=w417:dbl[], "best fit parameters"=→"profile fit":dbl[], "error out"=w424:errorcluster)  [unwired: 5 in, 3 out]
            n179 = Bundle(w445, "best nonlinear fit"=w417) -> (w448:cluster{dbl[], "best nonlinear fit":dbl[]})  [unwired: 1 in]
            n180 = Bundle(w445, w418) -> (w447:cluster{dbl[], dbl[]})  [unwired: 1 in]
            n181 = Build Array(w447, w448) -> (w450:cluster{dbl[], "best nonlinear fit":dbl[]}[])
            n182 = call <vilib>:"Clear Errors.vi"("error in (no error)"=w424) -> ("error out"=w427:errorcluster)  [unwired: 6 in]
            n183 = call <vilib>:"Goodness of Fit.vi"("Best Fit"=w417, "Y"=w418) -> ("R-square"=→"R-square":dbl)  [unwired: 6 in, 3 out]
            n184 = Absolute Value(x=w450) -> (abs(x)=→"Beam Profile":cluster{dbl[], "best nonlinear fit":dbl[]}[])
            n185 = property on="Beam Profile" class="XYGraph (strict)"(error in=w427, "Active Plot"=u32 0, "Plot.Plot Color"=w433, "Plot.Fill/Pt. Color"=w433, "Plot.Plot Interpolation"=u8 0 ("Plot.Line Style 2"), "Plot.Point Style"=u8 2 ("Plot.Point Style 2"), "Plot.Plot Name"="w_0", "Plot.Line Width"=u8 2, "Plot.Line Style"=u8 0) -> (error out=w435:errorcluster)  [unwired: 1 in, 1 out]
            n186 = property on="Beam Profile" class="XYGraph (strict)"(error in=w435, "Active Plot"=u32 1, "Plot.Plot Color"=w431, "Plot.Fill/Pt. Color"=w431, "Plot.Plot Interpolation"=u8 2 ("Plot.Line Style"), "Plot.Point Style"=u8 0, "Plot.Plot Name"="Z-Profile", "Plot.Line Style"=u8 0, "Plot.Line Width"=u8 1) -> (error out=w425:errorcluster)  [unwired: 1 in, 1 out]
            n187 = Bundle By Name(cluster=w456, "error"=w425) -> (w426:T10)
          }
          frame "CheckEndCondition" {
            w472 = 2  # axis Z
            # "Need to be refined, for future z positions automation."
            n188 = Unbundle By Name(w469) -> ("Scan#"=w470:i32, "File Header.Dimension"=w473:i32[])
            n189 = Index Array(array=w473, index=w472) -> (element=w471:i32)
            n190 = Greater Or Equal?(x=w470, y=w471) -> (x >= y?=w462:bool)
            n191 = Select(t=T15."Close" ("State"), s=w462, f=T15."PrepScanParams" ("State")) -> (s? t:f=w460:T15)
            n192 = Bundle By Name(cluster=w467, "State"=w460) -> (w461:T6)
            n193 = Enqueue Element(queue=w468, element=w461) -> ()  [unwired: 2 in, 3 out]
          }
          frame "Close" {
            # "Quit is done in QuitProg."
            n194 = Unbundle By Name(w487) -> ("ControlRefs.ProcCore_CtrlQueue"=w481:refnum<queue>, "ControlRefs.WriterSIG"=w486:refnum<queue>)
            n195 = Enqueue Element(queue=w492, element=T7 {"State"=enum."Close", "Params"=variant}) -> (error out=w475:errorcluster)  [unwired: 2 in, 2 out]
            n196 = Bundle By Name(cluster=T12 {"Command"=enum."SetWriterRef", "Params"=variant} ("element"), "Command"=ProcessStates."StopSave") -> (w480:T12)
            n197 = Bundle By Name(cluster=T12 {"Command"=enum."SetWriterRef", "Params"=variant} ("element"), "Command"=ProcessStates."SetWriterRef", "Params"=w486) -> (w489:T12)
            n198 = Enqueue Element(queue=w481, element=w480, error in (no error)=w475) -> (queue out=w479:refnum<queue>, error out=w478:errorcluster)  [unwired: 1 in, 1 out]
            n199 = Enqueue Element(queue=w479, element=w489, error in (no error)=w478) -> (error out=w477:errorcluster)  [unwired: 1 in, 2 out]
            n200 = property on="Quit" class="Bool (strict)"("Visible"=TRUE) -> ()  [unwired: 2 in, 2 out]
            n201 = call <vilib>:"Clear Errors.vi"("error in (no error)"=w477) -> ()  [unwired: 6 in, 1 out]
          }
          frame "Quit" {
            n202 = Unbundle By Name(w495) -> ("HighSpeed"=w494:dbl)
            n203 = Release Queue(queue=w503) -> (error out=w496:errorcluster)  [unwired: 2 in, 2 out]
            n204 = disable-structure shown="Enabled" {
              disable-tunnel: w497 -> [w521 _]
              disable-tunnel: w494 -> [w517 _]
              frame Enabled {
                # "Bad solution: have upper level jump out wait queue"
                n205 = Bundle By Name(cluster=T14 {"Line Start"=[], "Line End"=[], "HighSpeed"=0.0, "ScanSpeed"=0.0, "KeepStill(ms)"=0, "InstruParams"=[]} ("element"), "HighSpeed"=w517, "ScanSpeed"=nan) -> (w518:T14)
                n206 = Enqueue Element "! Not for setting speed"(queue=w521, element=w518) -> (error out=w519:errorcluster)  [unwired: 2 in, 2 out]
                n207 = call <vilib>:"Clear Errors.vi"("error in (no error)"=w519) -> ()  [unwired: 6 in, 1 out]
              }
              frame Disabled {
              }
            }
            n208 = property on="Quit" class="Bool (strict)"("Visible"=FALSE) -> ()  [unwired: 2 in, 2 out]
            n209 = Release Queue(queue=w513, error in (no error)=w496) -> (error out=w499:errorcluster)  [unwired: 1 in, 2 out]
            n210 = Enqueue Element(queue=w511, element=T7 {"State"=enum."QuitProg.", "Params"=variant}) -> (error out=w498:errorcluster)  [unwired: 2 in, 2 out]
            n211 = Generate User Event(user event=w508, event data cluster=cluster{bool} {TRUE} ("event data")) -> (user event out=w506:refnum<user-event>, error out=w505:errorcluster)  [unwired: 2 in]
            n212 = Destroy User Event(user event=w506, error in=w505) -> (error out=w501:errorcluster)
            n213 = Merge Errors(w501, w499, w498) -> (w500:errorcluster)
            n214 = Bundle By Name(cluster=w495, "error"=w500) -> (w502:T10)
          }
          frame "Refresh_BeamProfileSingle" {
            w523 = 2 ("index")
            # "Call command has to be push to the end not start of the queue."
            n215 = Unbundle By Name(w535) -> ("File Header"=w525:T5)
            n216 = disable-structure shown="Disabled" {
              disable-tunnel: w536 -> [w539 _]
              frame Disabled {
                n217 = Get Queue Status(queue=w539) -> (# pending remove=w538:i32)  [unwired: 2 in, 7 out]
                n218 = Equal To 0?(x=w538) -> (x = 0?=w537:bool)
                n219 = case shown="True" w537 {
                  frame False {
                  }
                  frame True {
                    n220 = One Button Dialog(message="Internal error:\nNothing in queue while refresh curves.") -> ()  [unwired: 1 in, 1 out]
                  }
                }
              }
              frame Enabled {
              }
            }
            n221 = Unbundle By Name(w525) -> ("Start Position"=w528:dbl[], "StepWidth"=w529:dbl[])
            n222 = Index Array(array=w533, index (row)="Scan#") -> (element=→"raw+fit":cluster{dbl[], dbl[]}[])  [unwired: 1 in]
            n223 = Index Array(array=w528, index=w523) -> (element=w530:dbl)
            n224 = Index Array(array=w529, index=w523) -> (element=w531:dbl)
            n225 = Multiply(x=w531, y="Scan#") -> (x*y=w526:dbl)
            n226 = Compound Arithmetic op=ADD(w530, w526) -> (→"z (mm)":dbl)
          }
        }
      }
      frame Error {
      }
    }
    "Iteration" <- w76
  }
  n227 = while {
    tunnel: w38 -> [w548]
    tunnel: w62 -> [w546]
    stop <- w547 stop-if-true
    n228 = event shown="[1] \"Quit\": Value Change;  Application Instance Close;  <Quit_UserEvent>: User Event;  Panel Close" {
      selector: w546 -> [_ _ _]
      dyn-events: _ -> [_ _ _]
      timeout: _ -> [_ _ _]
      tunnel: w548 -> [_ w552 w559]
      tunnel: [FALSE TRUE _] -> w547
      event Timeout {
        n229 = event-data() -> ()  [unwired: 1 in, 1 out]
      }
      event "Quit": Value Change; Application Instance Close; User Event; Panel Close {
        n230 = event-data() -> ()  [unwired: 1 in, 1 out]
        n231 = Enqueue Element(queue=w552, element=T6 {"State"=enum."Close", "Para."=variant}) -> (queue out=w553:refnum<queue>, error out=w551:errorcluster)  [unwired: 2 in, 1 out]
        n232 = call <vilib>:"Clear Errors.vi"("error in (no error)"=w551) -> ()  [unwired: 6 in, 1 out]
        n233 = property on="Quit" class="Bool (strict)"("Value"=FALSE ("Quit")) -> ()  [unwired: 2 in, 2 out]
        n234 = Enqueue Element(queue=w553, element=T6 {"State"=enum."Quit", "Para."=variant}) -> (error out=w555:errorcluster)  [unwired: 2 in, 2 out]
        n235 = call <vilib>:"Clear Errors.vi"("error in (no error)"=w555) -> ()  [unwired: 6 in, 1 out]
      }
      event "Scan#": Value Change {
        n236 = event-data() -> ()  [unwired: 1 in, 1 out]
        n237 = Enqueue Element At Opposite End(queue=w559, element=T6 {"State"=enum."Refresh_BeamProfileSingle", "Para."=variant}) -> ()  [unwired: 2 in, 3 out]
      }
    }
  }
  n238 = Unbundle By Name(w64) -> ("error"=w27:errorcluster)
  n239 = Merge Errors(w27, w29) -> (w28:errorcluster)
  n240 = Release Queue(queue=w46, error in (no error)=w28) -> (error out=w47:errorcluster)  [unwired: 1 in, 2 out]
  n241 = Release Queue(queue=w45, error in (no error)=w47) -> (error out=→"error out":errorcluster)  [unwired: 1 in, 2 out]
